vi "GetShutterStatus.vi"(8 "error in (no error)":errorcluster, 10 "Label":string, 11 "Laser_Oxxius in":refnum<class "Laser_Oxxius.lvclass">) -> (0 "error out":errorcluster, 2 "Value":bool, 3 "Laser_Oxxius out":refnum<class "Laser_Oxxius.lvclass">)   [LabVIEW 2020, in "Laser_Oxxius.lvlib" / "Laser_Oxxius.lvclass"]
uses:
  Laser_Oxxius.lvclass
  HAL Layer/Component/Laser/Laser/Laser.lvclass
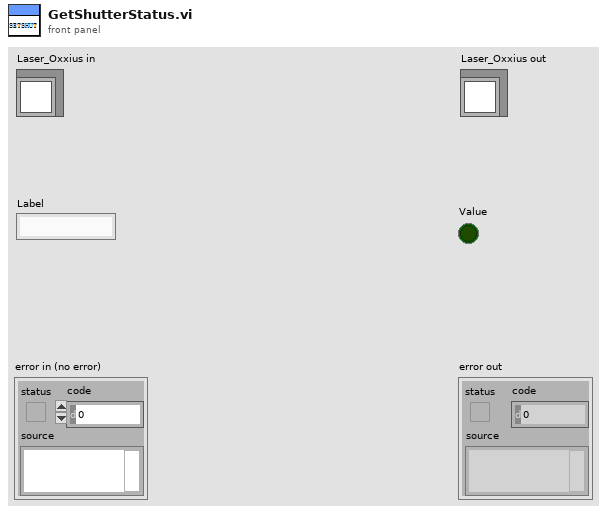
[diagram p1: front panel]
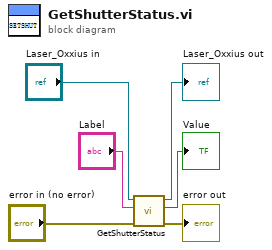
[diagram p0: block diagram]
diagram:
  n1 = call-parent "GetShutterStatus.vi"("error in (no error)"="error in (no error)", "Label"="Label", "Laser in"="Laser_Oxxius in") -> ("error out"=→"error out":errorcluster, "Value"=→"Value":bool, "Laser out"=→"Laser_Oxxius out":refnum<class "Laser_Oxxius.lvclass">)  [unwired: 6 in]
